vi "Null To Pretty String.vi"(7 "enable LabVIEW extensions? (T)":bool=TRUE, 8 "error in (no error)":errorcluster, 11 "JSON Datatype in":refnum<class "JSON Value.lvclass">) -> (0 "error out":errorcluster, 3 "Pretty Print String":string)   [LabVIEW 2016, in "JSON Value.lvclass"]
doc: "Pretty prints the given JSON data in an easier to read format."
uses:
  JSON Helper/JSON Value.lvclass
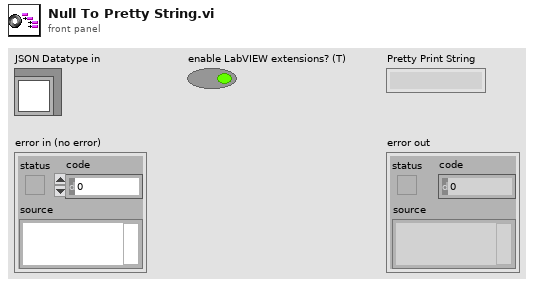
[diagram p1: front panel]
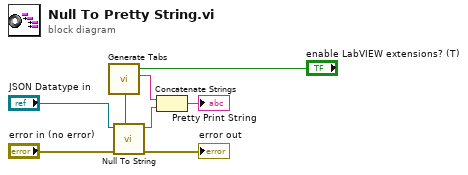
[diagram p0: block diagram]
diagram:
  n1 = call "Generate Tabs.vi"() -> ("Tabs"=w7:string)  [unwired: 10 in, 1 out]
  n2 = call "Null To String.vi"("enable LabVIEW extensions? (T)"="enable LabVIEW extensions? (T)", "error in (no error)"="error in (no error)", "JSON Datatype in"="JSON Datatype in") -> ("error out"=→"error out":errorcluster, "String"=w6:string)  [unwired: 7 in]
  n3 = Concatenate Strings(w7, w6) -> (→"Pretty Print String":string)
